vi "DI limits calc.vi"(6 "control":cluster{"invert":dbl, "time_const":dbl}={"invert"=0.0, "time_const"=100.0} {"time_const" min=-100000.0 max=100000.0 step=0.0010000000474974513; "invert" min=-100000.0 max=100000.0 step=0.0010000000474974513}, 7 "DI":bool) -> (0 "block":u32 format="%09b", 1 "Off":u32 format="%09b", 2 "On":u32 format="%09b", 3 "DIOUT":bool)   [LabVIEW 2019, in "Inputs.lvlib"]
uses:
  Inputs.lvlib
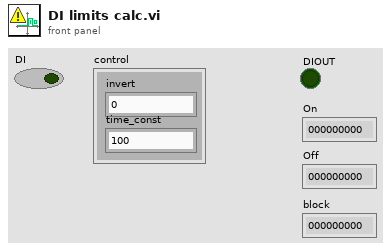
[diagram p1: front panel]
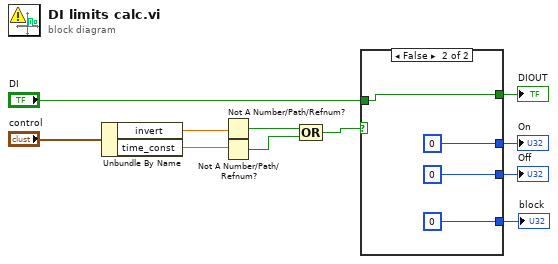
[diagram p0: block diagram]
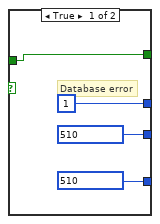
[diagram p2: hidden frame]
diagram:
  n1 = Unbundle By Name("control") -> ("invert"=w3:dbl, "time_const"=w2:dbl)
  n2 = Not A Number/Path/Refnum?(number/path/refnum=w3) -> (NaN/Path/Refnum?=w8:bool)
  n3 = Not A Number/Path/Refnum?(number/path/refnum=w2) -> (NaN/Path/Refnum?=w7:bool)
  n4 = Compound Arithmetic op=OR(w8, w7) -> (w6:bool)
  n5 = case shown="False" w6 {
    tunnel: [w15 w19] -> w11
    tunnel: "DI" -> [w15 w19]
    tunnel: [u32 1 u32 0] -> w10
    tunnel: [u32 510 u32 0] -> w9
    tunnel: [u32 510 u32 0] -> w5
    frame True {
      # "Database error"
    }
    frame False {
    }
  }
  "DIOUT" <- w11
  "On" <- w10
  "Off" <- w9
  "block" <- w5
